vi "Deadband.vi"(9 "deadband":dbl, 10 "value":dbl) -> (2 "ret value":dbl)   [LabVIEW 2016]
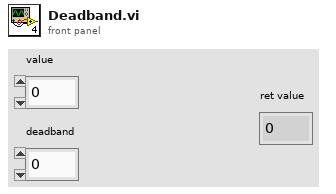
[diagram p1: front panel]
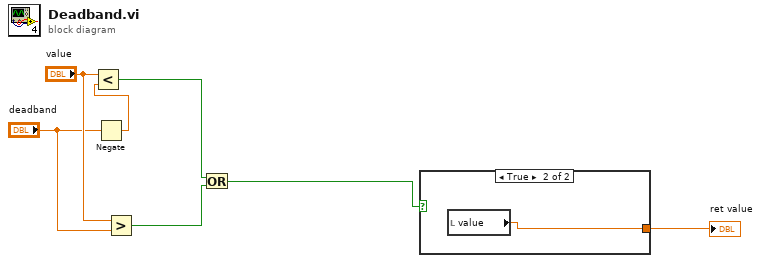
[diagram p0: block diagram]
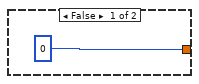
[diagram p2: hidden frame]
diagram:
  n1 = Negate(x="deadband") -> (-x=w7:dbl)
  n2 = Less?(x="value", y=w7) -> (x < y?=w3:bool)
  n3 = Greater?(x="value", y="deadband") -> (0:w2:bool)
  n4 = Or(x=w3, y=w2) -> (x .or. y?=w1:bool)
  n5 = case shown="True" w1 {
    tunnel: [0 w9] -> w4
    frame False {
    }
    frame True {
      n6 = local read "value"() -> (w9:dbl)
    }
  }
  "ret value" <- w4
